vi "Set Delay.vi"(8 "error in":errorcluster, 9 "Line":i32, 10 "PWM Delay":dbl format="%.3g", 11 "BNT_DAQmx-MCSV-DOPWM in":refnum<class "BNT_DAQmx-MCSV-DOPWM.lvclass">) -> (0 "error out":errorcluster, 3 "BNT_DAQmx-MCSV-DOPWM out":refnum<class "BNT_DAQmx-MCSV-DOPWM.lvclass">)   [LabVIEW 2020, in "BNT_DAQmx.lvlib" / "BNT_DAQmx-MCSV-DOPWM.lvclass"]
doc: "Set pulse delay at index."
uses:
  BNT_DAQmx-MCSV-DOPWM.lvclass
  C:/Users/holge/Documents/LVP/BNT/PGC/Packages/BNT_DAQmx/BNT_DAQmx-MCSV/BNT_DAQmx-MCSV.lvclass
  BNT_DAQmx-MCSV/BNT_DAQmx-MCSV.lvclass/BNT_DAQmx-MCSV.ctl
  BNT_DAQmx-MCSV-DOPWM.lvclass/BNT_DAQmx-MCSV-DOPWM.ctl
  CSPP_Core/Classes/CSPP_ProcessVariables/PVConnection/PVConnection.lvclass/PVConnection.ctl
  CSPP_Core/Classes/CSPP_ProcessVariables/ProcessVariable/PV.lvclass/PV.ctl
  CSPP_Core/Classes/CSPP_ProcessVariables/ProcessVariable/Write Data.vi
  CSPP_Core/Classes/CSPP_ProcessVariables/ProcessVariable/Write Error.vi
  CSPP_Core/Classes/CSPP_ProcessVariables/ProcessVariable/Write Quality.vi
  CSPP_Core/Classes/CSPP_ProcessVariables/ProcessVariable/Write status.vi
  CSPP_Core/Classes/CSPP_ProcessVariables/ProcessVariable/Write Timestamp.vi
  CSPP_Core/Classes/CSPP_ProcessVariables/ProcessVariable/PV.lvclass
  CSPP_Core/Classes/CSPP_ProcessVariables/PVConnection/PVConnection.lvclass
  BNT_DAQmx-MCSV/BNT_DAQmx-MCSV.lvclass
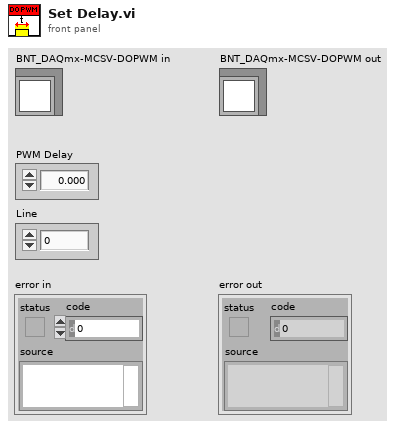
[diagram p1: front panel]
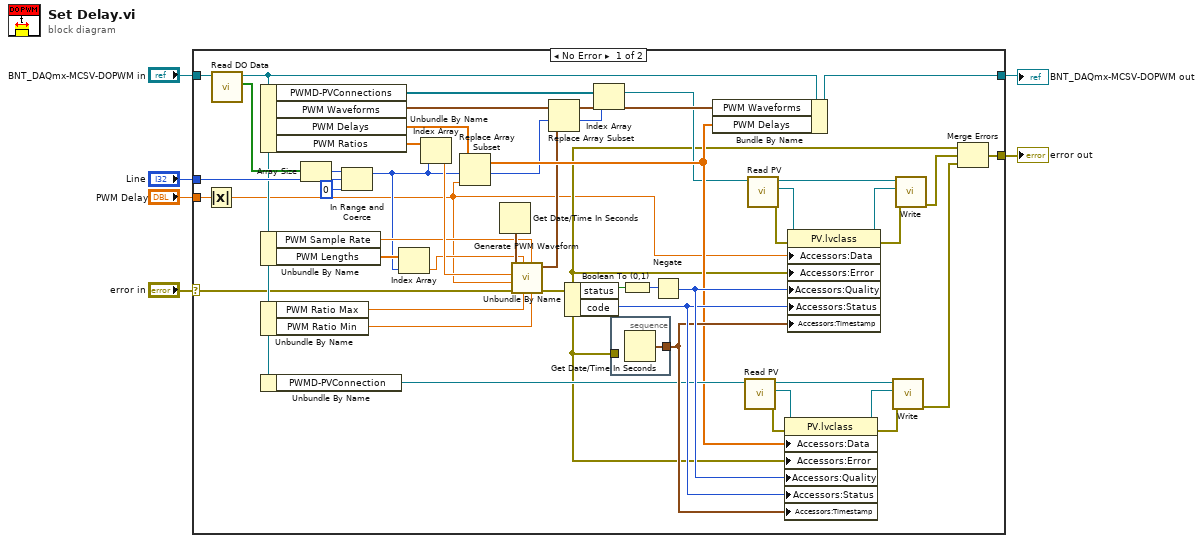
[diagram p0: block diagram]
diagram:
  n1 = case shown="No Error" "error in" {
    selector: "error in" -> [w19 w55]
    tunnel: [w49 w55] -> w2
    tunnel: [w47 w54] -> w1
    tunnel: "BNT_DAQmx-MCSV-DOPWM in" -> [w26 w54]
    tunnel: "PWM Delay" -> [w11 _]
    tunnel: "Line" -> [w22 _]
    frame No Error {
      n2 = Absolute Value(x=w11) -> (abs(x)=w7:dbl)
      n3 = call "Read DO Data.vi"("BNT_DAQmx-MCSV in"=w26) -> ("DO Data"=w25:bool[], "BNT_DAQmx-MCSV out"=w20:refnum<class "BNT_DAQmx-MCSV-DOPWM.lvclass">)  [unwired: 8 in, 1 out]
      n4 = Unbundle By Name(w20) -> ("PWMD-PVConnections"=w48:refnum<class "PVConnection.lvclass">[], "PWM Waveforms"=w35:waveform(dbl)[], "PWM Delays"=w36:dbl[], "PWM Ratios"=w21:dbl[])
      n5 = Unbundle By Name(w20) -> ("PWM Sample Rate"=w12:dbl[unit], "PWM Lengths"=w10:dbl[unit][])
      n6 = Unbundle By Name(w20) -> ("PWM Ratio Max"=w14:dbl, "PWM Ratio Min"=w13:dbl)
      n7 = Unbundle By Name(w20) -> ("PWMD-PVConnection"=w37:refnum<class "PVConnection.lvclass">)
      n8 = Array Size(array=w25) -> (size(s)=w24:i32)
      n9 = In Range and Coerce(upper limit=w24, x=w22, lower limit=0) -> (coerced(x)=w8:i32)  [unwired: 1 out]
      n10 = Index Array(array=w10, index=w8) -> (element=w9:dbl[unit])
      n11 = Index Array(array=w21, index=w8) -> (element=w15:dbl)
      n12 = Replace Array Subset(array=w36, new element=w7, index=w8) -> (w33:dbl[])
      n13 = Get Date/Time In Seconds() -> (seconds since 1Jan1904=w17:timestamp)
      n14 = call "Generate PWM Waveform.vi"("PWM Ratio Min"=w13, "PWM Sample Rate"=w12, "PWM Ratio Max"=w14, "PWM Length"=w9, "error in (no error)"=w19, "PWM Delay"=w7, "PWM Ratio"=w15, "Timestamp"=w17) -> ("error out"=w16:errorcluster, "PWM Waveform"=w18:waveform(dbl))  [unwired: 2 in]
      n15 = Replace Array Subset(array=w35, new element=w18, index=w8) -> (w34:waveform(dbl)[])
      n16 = Unbundle By Name(w16) -> ("status"=w51:bool, "code"=w40:i32)
      n17 = Index Array(array=w48, index=w8) -> (element=w32:refnum<class "PVConnection.lvclass">)
      n18 = stacked-sequence {
        tunnel: [w53] -> w39
        tunnel: w16 -> [_]
        frame #0 {
          n19 = Get Date/Time In Seconds() -> (seconds since 1Jan1904=w53:timestamp)
        }
      }
      n20 = Boolean To (0,1)(Boolean=w51) -> (0, 1=w52:i16)
      n21 = Negate(x=w52) -> (-x=w41:i16)
      n22 = Bundle By Name(cluster=w20, "PWM Waveforms"=w34, "PWM Delays"=w33) -> (w47:refnum<class "BNT_DAQmx-MCSV-DOPWM.lvclass">)
      n23 = call "Read PV.vi"("PVConnection in"=w37) -> ("error out"=w46:errorcluster, "PV"=w45:refnum<class "PV.lvclass">, "PVConnection out"=w44:refnum<class "PVConnection.lvclass">)  [unwired: 8 in]
      n24 = call "Read PV.vi"("PVConnection in"=w32) -> ("error out"=w27:errorcluster, "PV"=w28:refnum<class "PV.lvclass">, "PVConnection out"=w29:refnum<class "PVConnection.lvclass">)  [unwired: 8 in]
      n25 = property class="PV.lvclass"(reference=w45, error in=w46, "Accessors:Data"=w33, "Accessors:Error"=w16, "Accessors:Quality"=w41, "Accessors:Status"=w40, "Accessors:Timestamp"=w39) -> (reference out=w42:refnum<class "PV.lvclass">, error out=w43:errorcluster)
      n26 = property class="PV.lvclass"(reference=w28, error in=w27, "Accessors:Data"=w7, "Accessors:Error"=w16, "Accessors:Quality"=w41, "Accessors:Status"=w40, "Accessors:Timestamp"=w39) -> (reference out=w31:refnum<class "PV.lvclass">, error out=w30:errorcluster)
      n27 = call "Write.vi"("error in (no error)"=w43, "PV"=w42, "PVConnection in"=w44) -> ("error out"=w38:errorcluster)  [unwired: 6 in, 2 out]
      n28 = call "Write.vi"("error in (no error)"=w30, "PV"=w31, "PVConnection in"=w29) -> ("error out"=w50:errorcluster)  [unwired: 6 in, 2 out]
      n29 = Merge Errors(w16, w50, w38) -> (w49:errorcluster)
    }
    frame Error {
    }
  }
  "error out" <- w2
  "BNT_DAQmx-MCSV-DOPWM out" <- w1
